vi "Event Loop.vi"(8 "Dev Actor Refs":refnum<queue>, 9 "Dev Actor Events":refnum<queue>, 10 "Actor":refnum<class "Actor.lvclass">, 11 "Dev Actor Panel":refnum<class "Dev Panel.lvclass">) -> ()   [LabVIEW 2021, in "Dev Panel.lvclass"]
uses:
  Dev Panel.lvclass
  <vilib>/jettl/jettl/Actor/Actor/Actor.lvclass
  Dev Actor Events.ctl
  Dev Actor Refs.ctl
  Dev Panel.lvclass/Dev Panel.ctl
  <vilib>/jettl/jettl/Actor/Msgs/Destroy/Destroy Msg/Destroy Msg.lvclass
  C:/Program Files/National Instruments/LabVIEW 2021/vi.lib/jettl/jettl/Actor/Msg/Msg.lvclass
  Msgs/Pop Up/Pop Up Msg/Pop Up Msg.lvclass
  <vilib>/jettl/jettl/Actor/Msgs/Merge Error/Merge Error Msg/Merge Error Msg.lvclass
panel:
  out "String Indicator":string
  in  "Pop Up":bool
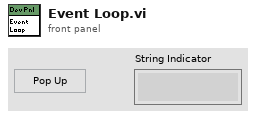
[diagram p1: front panel]
types:
  T1 = typedef "Dev Actor Events.ctl" = cluster{"Teardown":refnum<user-event>, "String Indicator":refnum<user-event>}
  T2 = typedef "Dev Actor Refs.ctl" = cluster{"Pop Up":refnum<vi>, "String Indicator":refnum<vi>}
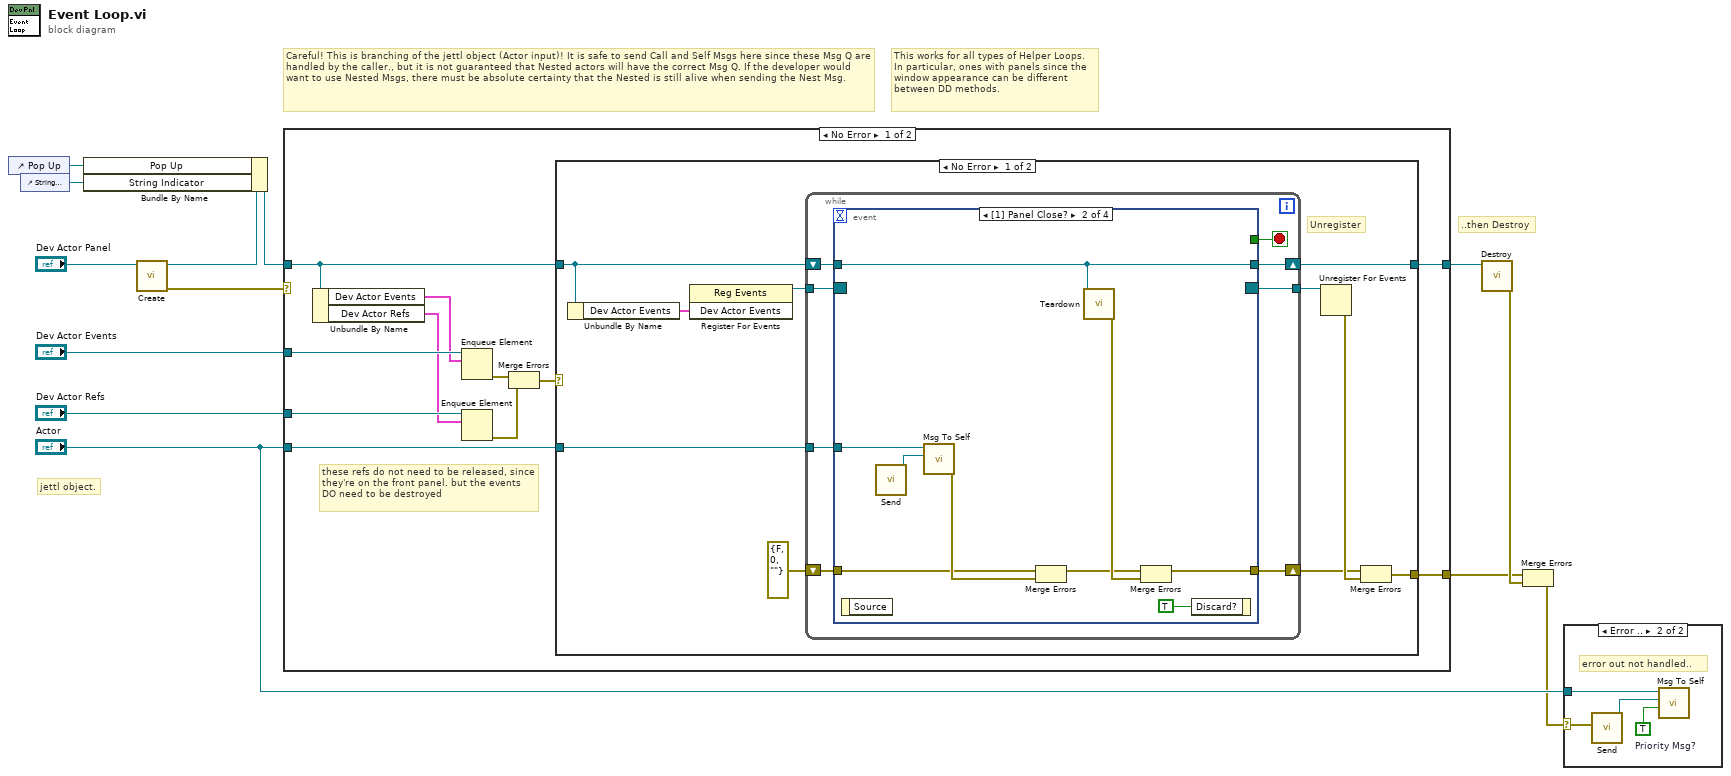
[diagram p0: block diagram]
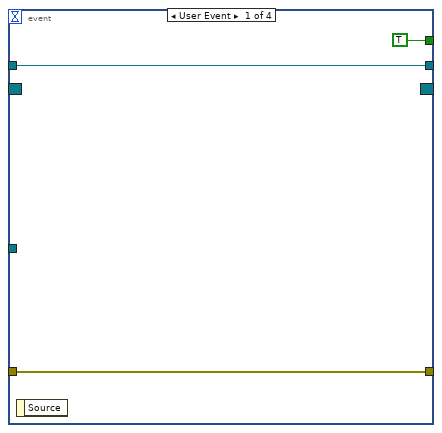
[diagram p3: hidden frame]
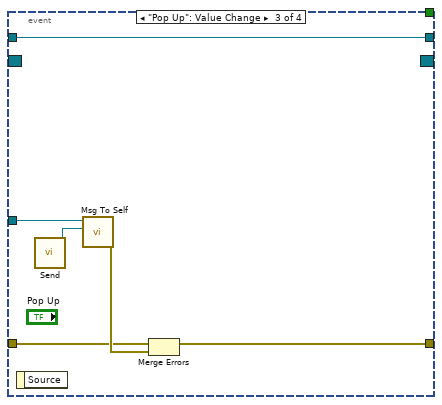
[diagram p4: hidden frame]
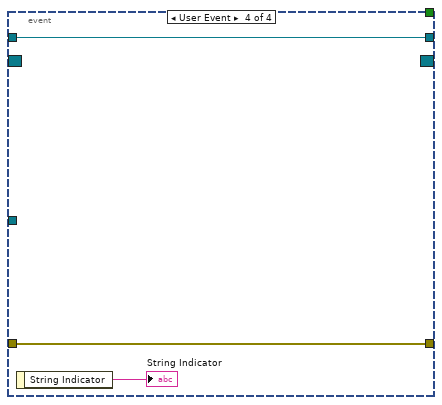
[diagram p5: hidden frame]
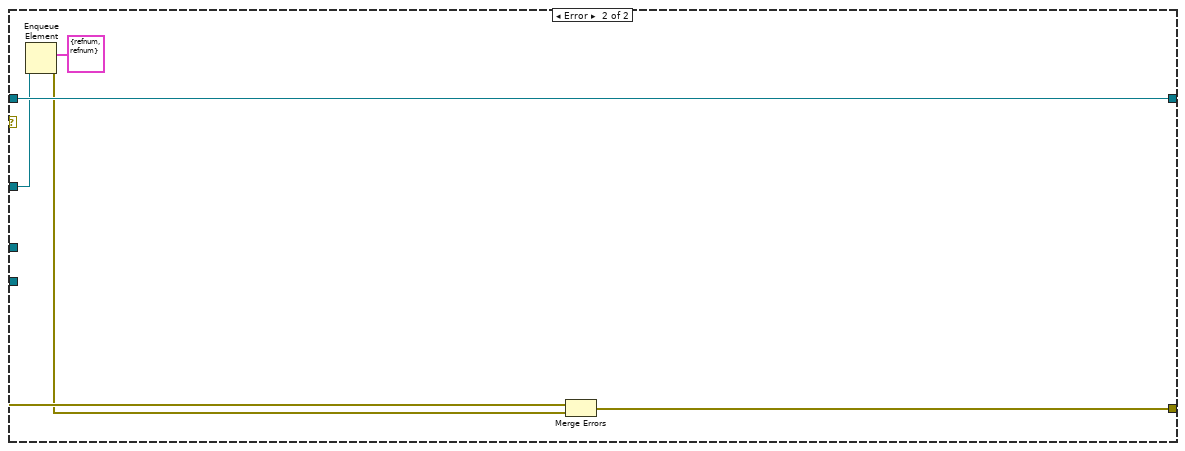
[diagram p7: hidden frame]
diagram:
  # "This works for all types of Helper Loops. In particular, ones with panels since the window appearance can be different between DD methods."
  # "..then Destroy"
  # "jettl object."
  # "Careful! This is branching of the jettl object (Actor input)! It is safe to send Call and Self Msgs here since these Msg Q are handled by the caller., but it is not guaranteed that Nested actors will have the correct Msg Q. If the developer would want to use Nested Msgs, there must be absolute certainty that the Nested is still alive when sending the Nest Msg."
  n1 = control-ref of="Pop Up"() -> (w4:refnum<vi>)
  n2 = control-ref of="String Indicator"() -> (w5:refnum<vi>)
  n3 = call "Create.vi"("Dev Actor Panel in"="Dev Actor Panel") -> ("error out"=w10:errorcluster, "Dev Actor Panel out"=w11:refnum<class "Dev Panel.lvclass">)  [unwired: 9 in]
  n4 = Bundle By Name(cluster=w11, "Pop Up"=w4, "String Indicator"=w5) -> (w6:refnum<class "Dev Panel.lvclass">)
  n5 = case shown="No Error" w10 {
    selector: w10 -> [_ w70]
    tunnel: "Actor" -> [w24 _]
    tunnel: [w23 w71] -> w13
    tunnel: w6 -> [w20 w71]
    tunnel: [w22 w67] -> w7
    tunnel: "Dev Actor Events" -> [w18 w69]
    tunnel: "Dev Actor Refs" -> [w19 _]
    frame No Error {
      # "these refs do not need to be released, since they're on the front panel. but the events DO need to be destroyed"
      n6 = Unbundle By Name(w20) -> ("Dev Actor Events"=w15:T1, "Dev Actor Refs"=w16:T2)
      n7 = Enqueue Element(queue=w18, element=w15) -> (error out=w21:errorcluster)  [unwired: 2 in, 2 out]
      n8 = Enqueue Element(queue=w19, element=w16) -> (error out=w17:errorcluster)  [unwired: 2 in, 2 out]
      n9 = Merge Errors(w21, w17) -> (w14:errorcluster)
      n10 = case shown="No Error" w14 {
        selector: w14 -> [_ w65]
        tunnel: w24 -> [w31 _]
        tunnel: [w30 w64] -> w23
        tunnel: [w28 w65] -> w22
        tunnel: w20 -> [w25 w64]
        frame No Error {
          # "Unregister"
          n11 = Unbundle By Name(w25) -> ("Dev Actor Events"=w32:T1)
          n12 = register-events ("Main Register for Events")(w32) -> (reference out=w33:refnum<event-registration>)  [unwired: 2 in, 1 out]
          n13 = while {
            tunnel: w31 -> [w39]
            shift-right: [w38] -> w30
            shift-left: w25 -> [w37]
            tunnel: w33 -> [w42]
            tunnel: [w40] -> w34
            shift-right: [w36] -> w26
            shift-left: errorcluster {"status"=FALSE, "code"=0, "source"=""} ("error out") -> [w35]
            stop <- w41 stop-if-true
            n14 = event "UI Events" shown="[1] Panel Close?" {
              selector: w42 -> [_ _ _ _]
              dyn-events: [_ _ _ _] -> w40
              timeout: _ -> [_ _ _ _]
              tunnel: [TRUE _ _ _] -> w41
              tunnel: w39 -> [_ w53 w59 _]
              tunnel: [w44 w49 w58 w63] -> w38
              tunnel: w37 -> [w44 w49 w58 w63]
              tunnel: [w43 w48 w57 w62] -> w36
              tunnel: w35 -> [w43 w50 w55 w62]
              event User Event {
                n15 = event-data() -> ()  [unwired: 1 in, 1 out]
              }
              event Panel Close? {
                n16 = event-data() -> ()  [unwired: 1 in, 1 out]
                n17 = call <vilib>:"Send.vi"() -> ("Destroy Msg out"=w52:refnum<class "Destroy Msg.lvclass">)  [unwired: 11 in]
                n18 = call-dynamic "Msg To Self.vi"("Msg"=w52, "Actor in"=w53) -> ("error out"=w51:errorcluster)  [unwired: 9 in]
                n19 = Merge Errors(w50, w51) -> (w46:errorcluster)
                n20 = call-dynamic "Teardown.vi"("Dev Actor Panel in"=w49) -> ("error out"=w47:errorcluster)  [unwired: 10 in]
                n21 = Merge Errors(w46, w47) -> (w48:errorcluster)
                n22 = event-data("Discard?"=TRUE) -> ()  [unwired: 1 in, 1 out]
              }
              event "Pop Up": Value Change {
                n23 = event-data() -> ()  [unwired: 1 in, 1 out]
                n24 = call <vilib>:"Send.vi"() -> ("Pop Up Msg out"=w60:refnum<class "Pop Up Msg.lvclass">)  [unwired: 11 in]
                n25 = call-dynamic "Msg To Self.vi"("Msg"=w60, "Actor in"=w59) -> ("error out"=w56:errorcluster)  [unwired: 9 in]
                n26 = Merge Errors(w55, w56) -> (w57:errorcluster)
              }
              event User Event {
                n27 = event-data() -> ("String Indicator"=→"String Indicator":string)  [unwired: 1 in]
              }
            }
          }
          n28 = Unregister For Events(event registration refnum=w34) -> (error out=w27:errorcluster)  [unwired: 1 in]
          n29 = Merge Errors(w26, w27) -> (w28:errorcluster)
        }
        frame Error {
        }
      }
    }
    frame Error {
      n30 = Enqueue Element(queue=w69, element=T1 {"Teardown"=refnum, "String Indicator"=refnum}) -> (error out=w66:errorcluster)  [unwired: 2 in, 2 out]
      n31 = Merge Errors(w70, w66) -> (w67:errorcluster)
    }
  }
  n32 = call "Destroy.vi"("Dev Actor Panel in"=w13) -> ("error out"=w8:errorcluster)  [unwired: 10 in]
  n33 = Merge Errors(w7, w8) -> (w1:errorcluster)
  n34 = case shown="Error .." w1 {
    selector: w1 -> [_ w73]
    tunnel: "Actor" -> [_ w75]
    frame No Error {
    }
    frame Error {
      w74 = TRUE  # Priority Msg?
      # "error out not handled.."
      n35 = call <vilib>:"Send.vi"("Error"=w73) -> ("Merge Error Msg out"=w72:refnum<class "Merge Error Msg.lvclass">)  [unwired: 10 in]
      n36 = call-dynamic "Msg To Self.vi"("Priority Msg?"=w74, "Msg"=w72, "Actor in"=w75) -> ()  [unwired: 8 in, 1 out]
    }
  }
